vi "Item.vi"(8 "error in (no error)":errorcluster, 10 "Index":i32, 11 "BufferedArray in":refnum<class "BufferedArray.lvclass">) -> (0 "error out":errorcluster, 1 "Item":refnum<class>, 3 "BufferedArray out":refnum<class "BufferedArray.lvclass">)   [LabVIEW 2013, in "LapDog.Collections.v1.Lists.Implementations.lvlib" / "BufferedArray.lvclass"]
doc: "Returns a copy of an item from the list at the given Index. An Index of -1 returns the last item in the list. If no item exists at the given Index error 510201 is returned."
uses:
  BufferedArray.lvclass
  BufferedArray.lvclass/BufferedArray.ctl
  LapDog.Collections.Common/LapDog.Collections.v1.Common.lvlib
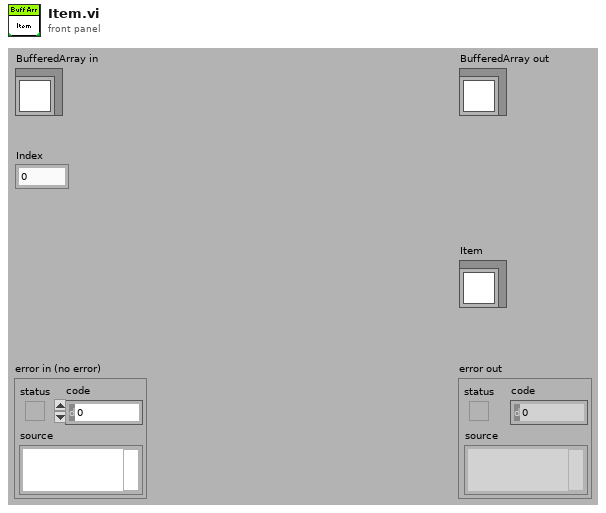
[diagram p1: front panel]
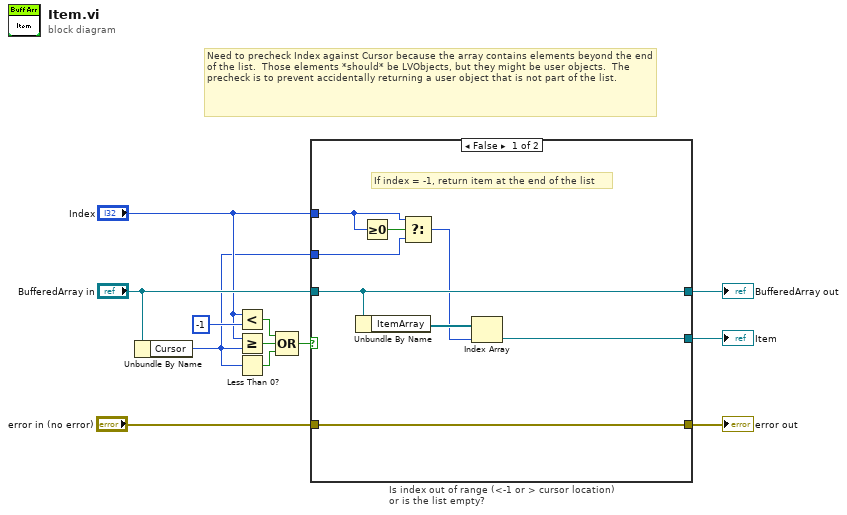
[diagram p0: block diagram]
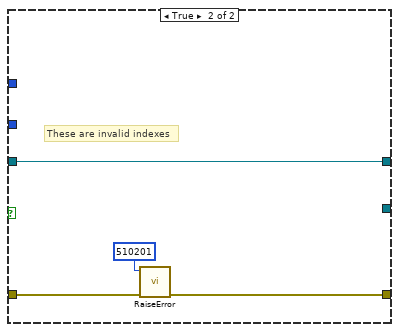
[diagram p2: hidden frame]
diagram:
  # "Need to precheck Index against Cursor because the array contains elements beyond the end of the list.  Those elements *should* be LVObjects, but they might be user objects.  The precheck is to prevent accidentally returning a user object that is not part of the list."
  n1 = Unbundle By Name("BufferedArray in") -> ("Cursor"=w3:i32)
  n2 = Less?(x="Index", y=-1) -> (x < y?=w1:bool)
  n3 = Greater Or Equal?(x="Index", y=w3) -> (x >= y?=w9:bool)
  n4 = Less Than 0?(x=w3) -> (x < 0?=w2:bool)
  n5 = Compound Arithmetic op=OR(w1, w9, w2) -> (w6:bool)
  n6 = case "Is index out of range (<-1 or > cursor location) or is the list empty?" shown="False" w6 {
    tunnel: "BufferedArray in" -> [w20 w24]
    tunnel: [w20 w24] -> w12
    tunnel: "Index" -> [w15 _]
    tunnel: [w19 _] -> w11
    tunnel: [w17 w21] -> w4
    tunnel: "error in (no error)" -> [w17 w22]
    tunnel: w3 -> [w13 _]
    frame False {
      # "If index = -1, return item at the end of the list"
      n7 = Unbundle By Name(w20) -> ("ItemArray"=w18:refnum<class>[])
      n8 = Greater Or Equal To 0?(x=w15) -> (x >= 0?=w16:bool)
      n9 = Select(t=w15, s=w16, f=w13) -> (s? t:f=w14:i32)
      n10 = Index Array(array=w18, index=w14) -> (element=w19:refnum<class>)
    }
    frame True {
      # "These are invalid indexes"
      n11 = call "RaiseError.vi"("error in (no error)"=w22, "Error Code"=510201) -> ("error out"=w21:errorcluster)  [unwired: 9 in]
    }
  }
  "error out" <- w4
  "BufferedArray out" <- w12
  "Item" <- w11
